vi "Connect.vi"(8 "error in (no error)":errorcluster, 10 "connectionList":string, 11 "SLSC Switch in":refnum<class "SLSC Switch.lvclass">) -> (0 "error out":errorcluster, 2 "switchActionArray":T1 {"relay action" items=["CloseRelay"=21, "OpenRelay"=20]}, 3 "SLSC Switch out":refnum<class "SLSC Switch.lvclass">)   [LabVIEW 2016, in "SLSC Switch.lvlib" / "SLSC Switch.lvclass"]
uses:
  SLSC Switch.lvclass
  Switch Action Processor/controls/SwitchAction Array.ctl
  Switch Action Processor/controls/Switch Action.ctl
  Relay/Relay Action.ctl
  Relay/Relay.lvclass
  Switch Action Processor/Switch Action Processor.lvclass
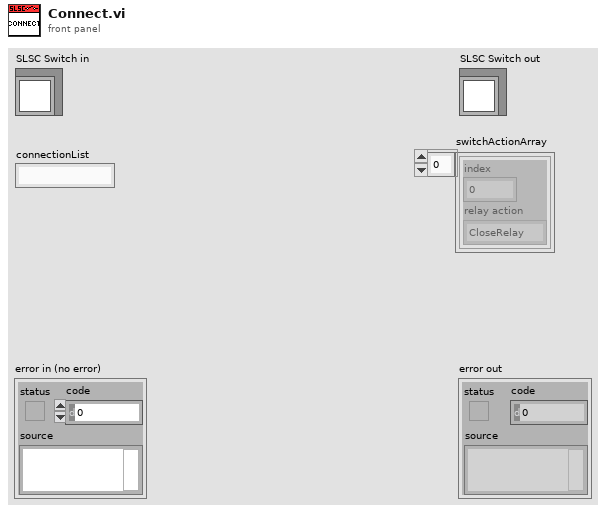
[diagram p1: front panel]
types:
  T1 = typedef "SLSC Switch.lvlib/Switch Action Processor.lvclass/SwitchAction Array.ctl" = T2[]
  T2 = typedef "SLSC Switch.lvlib/Switch Action Processor.lvclass/Switch Action.ctl" = cluster{"index":i32, "relay action":T3}
  T3 = typedef "SLSC Switch.lvlib/Relay.lvclass/Relay Action.ctl" = u32
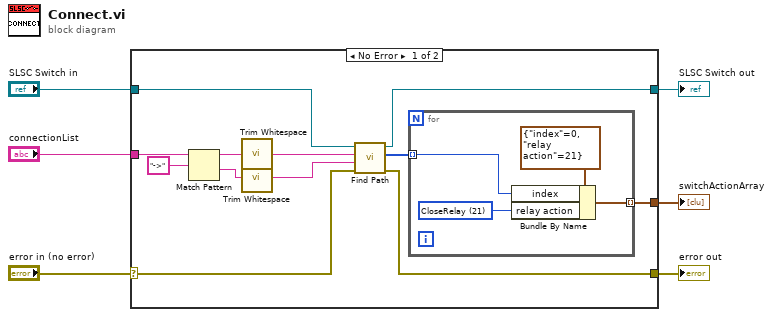
[diagram p0: block diagram]
diagram:
  n1 = case shown="No Error" "error in (no error)" {
    selector: "error in (no error)" -> [w11 w24]
    tunnel: [w10 w24] -> w5
    tunnel: [w7 w23] -> w3
    tunnel: "SLSC Switch in" -> [w12 w23]
    tunnel: "connectionList" -> [w17 _]
    tunnel: [w8 _] -> w1
    frame No Error {
      n2 = Match Pattern(string=w17, regular expression="->") -> (before substring=w16:string, after substring=w15:string)  [unwired: 1 in, 2 out]
      n3 = call <vilib>:"Trim Whitespace.vi"("string"=w16) -> ("trimmed string"=w13:string)  [unwired: 1 in]
      n4 = call <vilib>:"Trim Whitespace.vi"("string"=w15) -> ("trimmed string"=w14:string)  [unwired: 1 in]
      n5 = call "Find Path.vi"("error in (no error)"=w11, "channel 2"=w14, "channel 1"=w13, "SLSC Switch in"=w12) -> ("error out"=w10:errorcluster, "Relay Indexes"=w9:i32[], "SLSC Switch out"=w7:refnum<class "SLSC Switch.lvclass">)  [unwired: 5 in]
      n6 = for {
        tunnel: w9 -> [w22] mode=indexing
        tunnel: [w21] -> w8 mode=indexing
        w19 = T3 21 items=["CloseRelay"=21, "OpenRelay"=20] ("relay action")
        n7 = Bundle By Name(cluster=T2 {"index"=0, "relay action"=21} ("Switch Action"), "index"=w22, "relay action"=w19) -> (w21:T2)
      }
    }
    frame Error {
    }
  }
  "error out" <- w5
  "SLSC Switch out" <- w3
  "switchActionArray" <- w1
